vi "clLabview_md5.vi"() -> ()   [LabVIEW 2021, in "vi_lib.lvlib" / "clLabview.lvclass"]
uses:
  clLabview.lvclass
  clLabview.lvclass/clLabview.ctl
panel:
  out "source":string
  out "return vale 7":i32
  out "return vale 6":i32
  out "return vale 5":i32
  out "return vale 4":i32
  out "return vale 3":i32
  out "return vale 2":i32
  out "return vale":i32
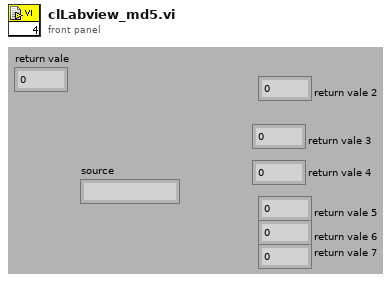
[diagram p1: front panel]
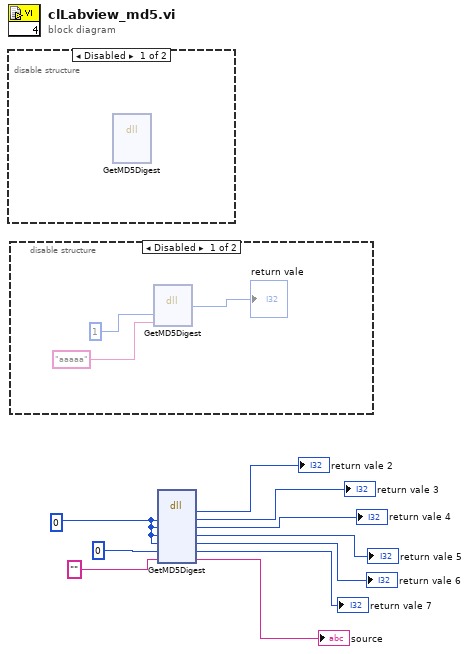
[diagram p0: block diagram]
diagram:
  w10 = u32 0 ("v1")
  n1 = disable-structure shown="Disabled" {
    frame Disabled {
      n2 = dll-call lib="LabVIEW" fn="GetMD5Digest"() -> ()  [unwired: 5 in, 7 out]
    }
    frame Enabled {
    }
  }
  n3 = disable-structure shown="Disabled" {
    frame Disabled {
      n4 = dll-call lib="LabVIEW" fn="GetMD5Digest"("size"=1 ("arg2"), "source"="aaaaa") -> ("return vale"=→"return vale":i32)  [unwired: 4 in, 3 out]
    }
    frame Enabled {
    }
  }
  n5 = dll-call lib="LabVIEW" fn="GetMD5Digest"("v1"=w10, "v2"=w10, "v3"=w10, "v4"=w10, "size"=0, "source"="") -> ("return vale"=→"return vale 2":i32, "v1"=→"return vale 3":u32, "v2"=→"return vale 4":i32, "v3"=→"return vale 5":i32, "v4"=→"return vale 6":i32, "size"=→"return vale 7":i32, "source"=→"source":string)  [unwired: 3 in, 2 out]
